vi "test.vi"   [LabVIEW 2021]
uses:
  FirstXNode .xnode
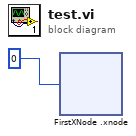
[diagram p0: block diagram]
diagram:
  n1 = xnode "FirstXNode .xnode"(0) -> ()  [unwired: 1 out]
